vi "ProcessImage.vi"(4 "Range":cluster{"Lower value":sgl, "Upper value":sgl}={"Lower value"=241.0, "Upper value"=255.0} {"Upper value" format="%.2f"; "Lower value" format="%.2f"}, 6 "New Image":T1, 7 "Pixel Measurements":T3[](array[typedef])=[35, 4, 5, 6, 7] items=["Center of Mass X", "Center of Mass Y", "First Pixel X", "First Pixel Y", "Bounding Rect Left", "Bounding Rect Top", "Bounding Rect Right", "Bounding Rect Bottom", "Max Feret Diameter Start X", "Max Feret Diameter Start Y", "Max Feret Diameter End X", "Max Feret Diameter End Y", "Max Horiz. Segment Length Left", "Max Horiz. Segment Length Right", "Max Horiz. Segment Length Row", "-", "Bounding Rect Width", "Bounding Rect Height", "Bounding Rect Diagonal", "Perimeter", "Convex Hull Perimeter", "Holes' Perimeter", "Max Feret Diameter", "Equivalent Ellipse Major Axis", "Equivalent Ellipse Minor Axis", "Equivalent Ellipse Minor Axis (Feret)", "Equivalent Rect Long Side", "Equivalent Rect Short Side", "Equivalent Rect Diagonal", "Equivalent Rect Short Side (Feret)", "Average Horiz. Segment Length", "Average Vert. Segment Length", "Hydraulic Radius", "Waddel Disk Diameter", "-", "Area", "Holes' Area", "Particle & Holes' Area", "Convex Hull Area", "Image Area", "-", "Number of Holes", "Number of Horiz. Segments", "Number of Vert. Segments", "-", "Orientation", "Max Feret Diameter Orientation", "-", "% Area/Image Area", "% Area/(Particle & Holes' Area)", "Ratio of Equivalent Ellipse Axes", "Ratio of Equivalent Rect Sides", "-", "Elongation Factor", "Compactness Factor", "Heywood Circularity Factor", "Type Factor", "-", "Sum X", "Sum Y", "Sum XX", "Sum XY", "Sum YY", "Sum XXX", "Sum XXY", "Sum XYY", "Sum YYY", "-", "Moment of Inertia XX", "Moment of Inertia XY", "Moment of Inertia YY", "Moment of Inertia XXX", "Moment of Inertia XXY", "Moment of Inertia XYY", "Moment of Inertia YYY", "Norm. Moment of Inertia XX", "Norm. Moment of Inertia XY", "Norm. Moment of Inertia YY", "Norm. Moment of Inertia XXX", "Norm. Moment of Inertia XXY", "Norm. Moment of Inertia XYY", "Norm. Moment of Inertia YYY", "Hu Moment 1", "Hu Moment 2", "Hu Moment 3", "Hu Moment 4", "Hu Moment 5", "Hu Moment 6", "Hu Moment 7"], 9 "Operation":T2(ring)=enum."Erode", 10 "Particle Count Limit":dbl=2.0, 11 "Refnum in":T1) -> (1 "Numeric":dbl, 2 "Particles":i32, 3 "Refnum out":T1(plugin-control))   [LabVIEW 2016]
uses:
  <vilib>/vision/Image Controls.llb/IMAQ Image.ctl
  <vilib>/Rock Robotics/Network Tables/NT Read Number.vi
  <vilib>/vision/NI_Vision_Development_Module.lvlib
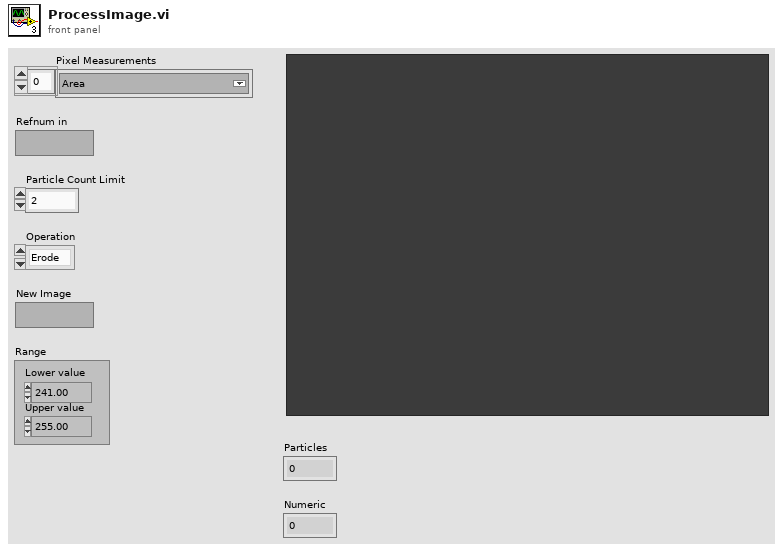
[diagram p1: front panel]
types:
  T1 = typedef "IMAQ Image.ctl" = refnum<image>
  T2 = enum32{"AutoM", "Close", "Dilate", "Erode", "Gradient", "Gradient in", "Gradient out", "HitMiss", "Open", "PClose", "POpen", "Thick", "Thin"}
  T3 = typedef "Particle Parameters" = i32
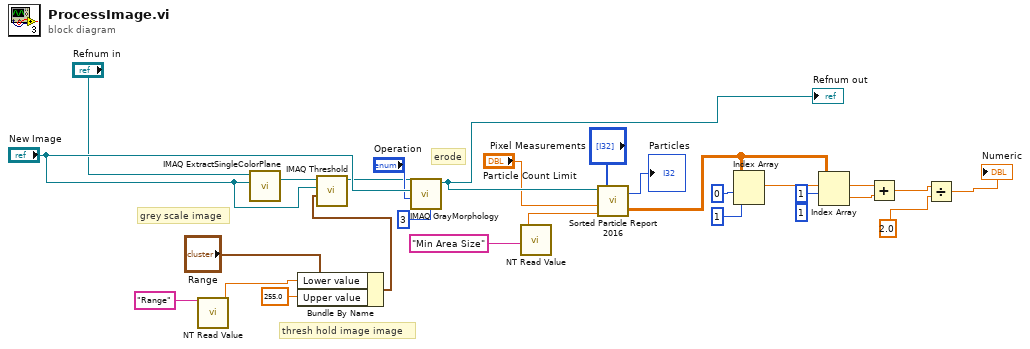
[diagram p0: block diagram]
diagram:
  # "erode"
  # "thresh hold image image"
  # "grey scale image"
  n1 = call-poly <vilib>:"NT Read Value.vi"("Name"="Range") -> ("Numeric"=w17:dbl)  [unwired: 9 in, 1 out]
  n2 = call "IMAQ ExtractSingleColorPlane"("Image Dst"="New Image", "Image Src"="Refnum in") -> ("Image Dst Out"=w1:T1)  [unwired: 8 in, 1 out]
  n3 = Bundle By Name(cluster="Range", "Lower value"=w17, "Upper value"=sgl 255.0) -> (w19:cluster{"Lower value":sgl, "Upper value":sgl})
  n4 = call "IMAQ Threshold"("Range"=w19, "Image Dst"="New Image", "Image Src"=w1) -> ("Image Dst Out"=w15:T1)  [unwired: 7 in, 1 out]
  n5 = call "IMAQ GrayMorphology"("Number of iterations (1)"=3, "Operation"="Operation", "Image Dst"="New Image", "Image Src"=w15) -> ("Image Dst Out"=w27:T1)  [unwired: 6 in, 1 out]
  "Refnum out" <- w27
  n6 = call-poly <vilib>:"NT Read Value.vi"("Name"="Min Area Size") -> ("Numeric"=w21:dbl)  [unwired: 9 in, 1 out]
  n7 = call "Sorted Particle Report 2016.vi"("Min Area Size %"=w21, "Particle Count Limit"="Particle Count Limit", "Pixel Measurements"="Pixel Measurements", "Image in"=w27) -> ("Sorted Data"=w10:dbl[][], "Particles"=→"Particles":i32)
  n8 = Index Array(array=w10, index (row)=0, index (col)=1 ("disabled index (col)")) -> (element=w12:dbl)
  n9 = Index Array(array=w10, index (row)=1, index (col)=1 ("disabled index (col)")) -> (element=w11:dbl)
  n10 = Add(x=w12, y=w11) -> (x+y=w5:dbl)
  n11 = Divide(x=w5, y=2.0) -> (x/y=→"Numeric":dbl)
